vi "Add Channel to Objects.vi"(8 "error in":errorcluster, 9 "Add? (T)":bool=TRUE, 10 "Line Item in":T1, 11 "Objects in":T4) -> (0 "error out":errorcluster, 2 "Line Index":i32)   [LabVIEW 2015, in "UI Reference editor node.lvclass"]
doc: "This VI adds the channel to the configuration Objects, and links the tag and the channel in the engine."
uses:
  UI Reference editor node.lvclass
  <vilib>/NI/DCAF/Tag Editor Core/Table API/Table Manager/object ref.ctl
  <vilib>/NI/DCAF/Tag Editor Core/Configuration Editor/Classes/Engine Parent/Engine Parent Editor Node.lvclass
  <vilib>/NI/DCAF/Tag Editor Core/Configuration Editor/Classes/Module editor node/module editor node.lvclass
  Mappings.ctl
  <vilib>/NI/Tag Bus Module Framework/channel/TBM channel.lvclass
  module/configuration/Line.ctl
  Map.ctl
  module/configuration/UI Reference configuration.lvclass
  <vilib>/NI/Configuration Framework/serializable configuration/NISE_CEF_serializable configuration.lvclass/NISE_CEF_serializable configuration.ctl
  <vilib>/Utility/LVClass/Get LV Class Name.vi
  <vilib>/NI/Configuration Framework/error generator/NISE_error generator.vi
  <vilib>/NI/Configuration Framework/serializable configuration/NISE_CEF_serializable configuration.lvclass
  <vilib>/NI/DCAF/Tag Editor Core/Table API/Table Manager/Table Manager.lvclass
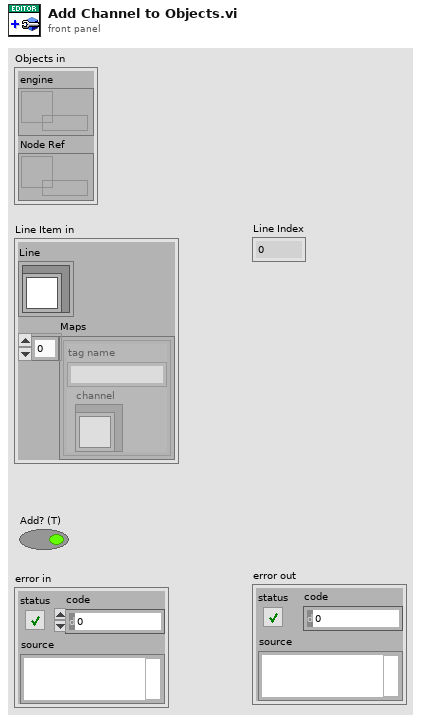
[diagram p1: front panel]
types:
  T1 = typedef "UI Reference editor node.lvclass/Mappings.ctl" = cluster{"Line":T2, "Maps":T3[]}
  T2 = typedef "UI Reference configuration.lvclass/Line.ctl" = cluster{"channel":refnum<class "TBM channel.lvclass">}
  T3 = typedef "UI Reference editor node.lvclass/Map.ctl" = cluster{"channel":refnum<class "TBM channel.lvclass">, "tag name":string}
  T4 = typedef "Table Manager.lvlib/Table Manager.lvclass/object ref.ctl" = cluster{"engine":refnum<data-value>, "Node Ref":refnum<data-value>}
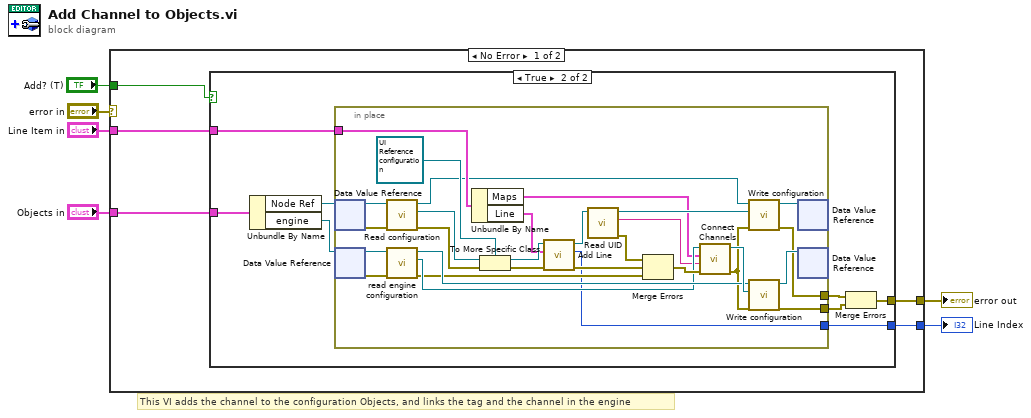
[diagram p0: block diagram]
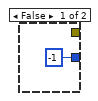
[diagram p2: hidden frame]
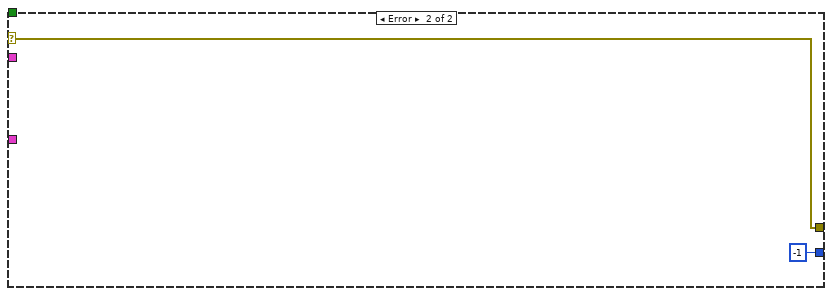
[diagram p3: hidden frame]
diagram:
  # "This VI adds the channel to the configuration Objects, and links the tag and the channel in the engine"
  n1 = case shown="No Error" "error in" {
    selector: "error in" -> [_ w51]
    tunnel: "Objects in" -> [w11 _]
    tunnel: "Line Item in" -> [w10 _]
    tunnel: "Add? (T)" -> [w9 _]
    tunnel: [w8 w51] -> w2
    tunnel: [w7 -1 ("Line Index")] -> w1
    frame No Error {
      n2 = case shown="True" w9 {
        tunnel: [_ w18] -> w8
        tunnel: w10 -> [_ w20]
        tunnel: w11 -> [_ w19]
        tunnel: [-1 ("Line Index") w13] -> w7
        frame False {
        }
        frame True {
          n3 = Unbundle By Name(w19) -> ("Node Ref"=w17:refnum<data-value>, "engine"=w16:refnum<data-value>)
          n4 = in-place {
            in-place-border: w20 -> [w49]
            in-place-border: [w36] -> w15
            in-place-border: [w34] -> w14
            in-place-border: [w22] -> w13
            n5 = in-place-dvr #1(w17) -> (w43:refnum<class "module editor node.lvclass">, w35:errorcluster)
            n6 = in-place-dvr #2(w16) -> (w33:refnum<class "Engine Parent Editor Node.lvclass">, w32:errorcluster)
            n7 = call-dynamic "Read configuration.vi"("error in"=w35, "NISE_CEF_serializable node in"=w43) -> ("error out"=w37:errorcluster, "configuration"=w38:refnum<class "NISE_CEF_serializable configuration.lvclass">, "NISE_CEF_serializable node out"=w42:refnum<class "module editor node.lvclass">)  [unwired: 7 in]
            n8 = call <vilib>:"read engine configuration.vi"("error in"=w32, "Engine Parent Editor Node in"=w33) -> ("error out"=w29:errorcluster, "engine configuration"=w30:refnum<class "engine configuration.lvclass">, "Engine Parent Editor Node out"=w31:refnum<class "Engine Parent Editor Node.lvclass">)  [unwired: 7 in]
            n9 = Unbundle By Name(w49) -> ("Maps"=w25:T3[], "Line"=w24:T2)
            n10 = To More Specific Class(target class=refnum<class "UI Reference configuration.lvclass"> refnum ("tag bus configurable plugin module configuration in"), reference=w38, error in=w37) -> (specific class reference=w47:refnum<class "UI Reference configuration.lvclass">, error out=w46:errorcluster)
            n11 = call "Add Line.vi"("error in"=w46, "Line"=w24, "UI Reference configuration in"=w47) -> ("error out"=w45:errorcluster, "Line Index"=w22:i32, "UI Reference configuration out"=w28:refnum<class "UI Reference configuration.lvclass">)  [unwired: 6 in]
            n12 = call <vilib>:"Read UID.vi"("configuration in"=w28) -> ("error out"=w21:errorcluster, "instance id"=w27:string, "configuration out"=w26:refnum<class "UI Reference configuration.lvclass">)  [unwired: 8 in]
            n13 = Merge Errors(w21, w45, w29) -> (w44:errorcluster)
            n14 = call "Connect Channels.vi"("error in (no error)"=w44, "instance id"=w27, "Maps"=w25, "Engine Configuration in"=w30) -> ("error out"=w23:errorcluster, "Engine Configuration out"=w39:refnum<class "engine configuration.lvclass">)  [unwired: 6 in]
            n15 = call-dynamic "Write configuration.vi"("error in"=w23, "configuration"=w26, "NISE_CEF_serializable node in"=w42) -> ("error out"=w34:errorcluster, "NISE_CEF_serializable node out"=w41:refnum<class "module editor node.lvclass">)  [unwired: 7 in]
            n16 = call-dynamic "Write configuration.vi"("error in"=w23, "configuration"=w39, "NISE_CEF_serializable node in"=w31) -> ("error out"=w36:errorcluster, "NISE_CEF_serializable node out"=w40:refnum<class "Engine Parent Editor Node.lvclass">)  [unwired: 7 in]
            n17 = in-place-dvr #1(w41) -> ()  [unwired: 2 out]
            n18 = in-place-dvr #2(w40) -> ()  [unwired: 2 out]
          }
          n19 = Merge Errors(w14, w15) -> (w18:errorcluster)
        }
      }
    }
    frame Error {
    }
  }
  "error out" <- w2
  "Line Index" <- w1
